vi "RPC.vi"(0 "mbed_LVLibrary.lvlib:HTTPRPC.lvclass":refnum<class "HTTPRPC.lvclass">, 5 "Name":string, 7 "method":string, 9 "Args":string[](array[string]), 11 "error in (no error)":errorcluster) -> (4 "mbed_LVLibrary.lvlib:HTTPRPC.lvclass 2":refnum<class "HTTPRPC.lvclass">, 8 "RPC Result":string, 15 "error out":errorcluster)   [LabVIEW 2011, in "mbed_LVLibrary.lvlib" / "HTTPRPC.lvclass"]
uses:
  HTTPRPC.lvclass
  HTTPRPC.lvclass/HTTPRPC.ctl
  mbed/mbed.lvclass
  <vilib>/wsapi/NI_WebServices.lvlib
panel:
  out "Data Returned from HTTP Server":string
  out "The TCP request":string
  out "The RPC string":string
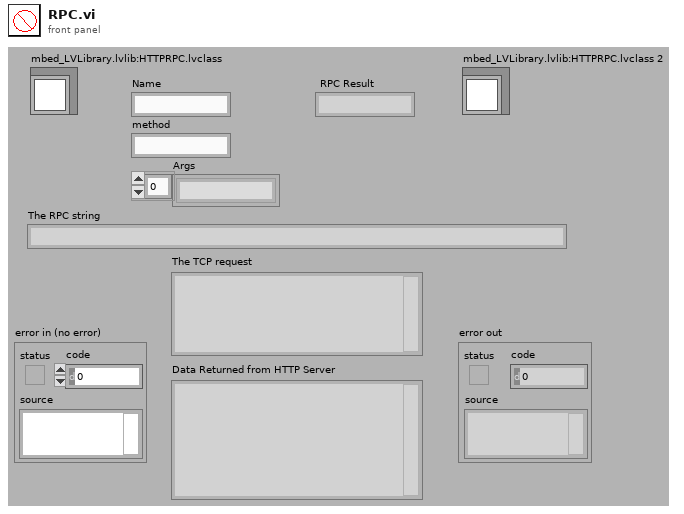
[diagram p1: front panel]
types:
  T1 = enum16{"Standard", "Buffered", "CRLF", "Immediate"}
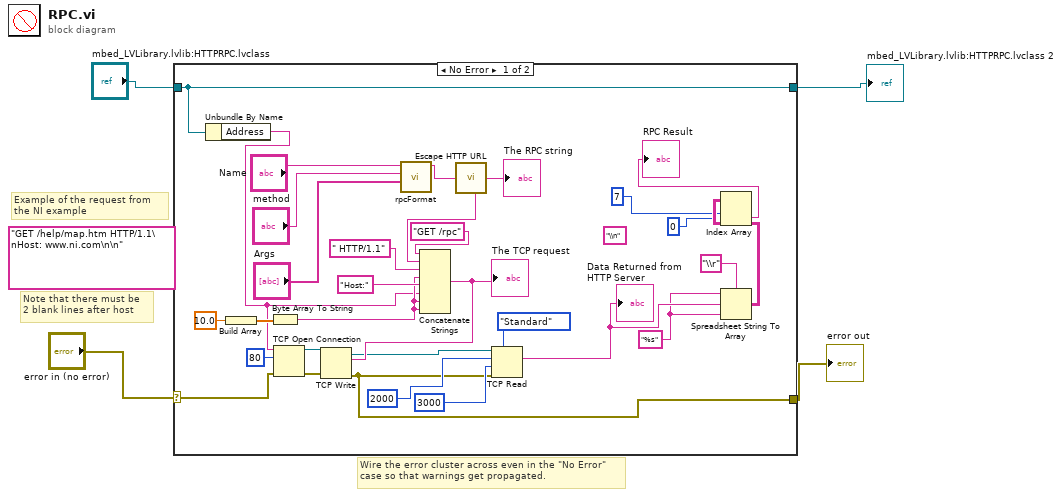
[diagram p0: block diagram]
diagram:
  (unwired) "GET /help/map.htm HTTP/1.1\nHost: www.ni.com\n\n" ("data in")
  # "Note that there must be \n2 blank lines after host"
  # "Example of the request from the NI example"
  # "Wire the error cluster across even in the \"No Error\"\ncase so that warnings get propagated."
  n1 = case shown="No Error" "error in (no error)" {
    selector: "error in (no error)" -> [w20 w36]
    tunnel: [w5 w36] -> w3
    tunnel: [w10 w35] -> w1
    tunnel: "mbed_LVLibrary.lvlib:HTTPRPC.lvclass" -> [w10 w35]
    frame No Error {
      w17 = "%s" ("format string")
      (unwired) "\\n" ("delimiter (Tab)")
      n2 = Unbundle By Name(w10) -> ("Address"=w23:string)
      n3 = Build Array(10.0 ("element")) -> (w29:dbl[])
      n4 = Byte Array To String(unsigned byte array=w29) -> (string=w27:string)
      n5 = TCP Open Connection(address=w23, remote port or service name=u16 80, error in (no error)=w20) -> (connection ID=w24:refnum<k5>, error out=w21:errorcluster)  [unwired: 2 in]
      n6 = call "rpcFormat.vi"("Args"="Args", "method"="method", "Name"="Name") -> ("The RPC string"=w6:string)  [unwired: 8 in]
      n7 = call <vilib>:"Escape HTTP URL.vi"("unescaped string in"=w6) -> ("escaped string out"=w7:string)
      "The RPC string" <- w7
      n8 = Concatenate Strings("GET /rpc" ("string"), w7, " HTTP/1.1" ("string"), w27, "Host:" ("string"), w23, w27, w27) -> (w30:string)
      "The TCP request" <- w30
      n9 = TCP Write(connection ID=w24, data in=w30, error in (no error)=w21) -> (connection ID out=w11:refnum<k5>, error out=w5:errorcluster)  [unwired: 1 in, 1 out]
      n10 = TCP Read(connection ID=w11, bytes to read=2000, error in (no error)=w5, 7:T1."Standard" ("mode (standard)"), 9:3000 ("timeout ms (25000)")) -> (data out=w18:string)  [unwired: 2 out]
      "Data Returned from HTTP Server" <- w18
      n11 = Spreadsheet String To Array(delimiter (Tab)="\\r", format string=w17, spreadsheet string=w18, array type (2D Dbl)=w17) -> (array=w15:string[][])
      n12 = Index Array(array=w15, index (row)=7, index (col)=0 ("disabled index (col)")) -> (element=→"RPC Result":string)
    }
    frame Error {
    }
  }
  "error out" <- w3
  "mbed_LVLibrary.lvlib:HTTPRPC.lvclass 2" <- w1
